vi "START ADD USER.vi"(10 "REFERENCES":T2, 11 "USER INFO IN":T1) -> (2 "User Image":T3, 3 "USER INFO OUT":T1)   [LabVIEW 2019]
uses:
  <vilib>/vision/Image Controls.llb/IMAQ Image.ctl
  Controls/References Cluster.ctl
  <vilib>/userDefined/High Color/IMAQdx.ctl
  Controls/Custom Calendar/Custom Calendar.xctl
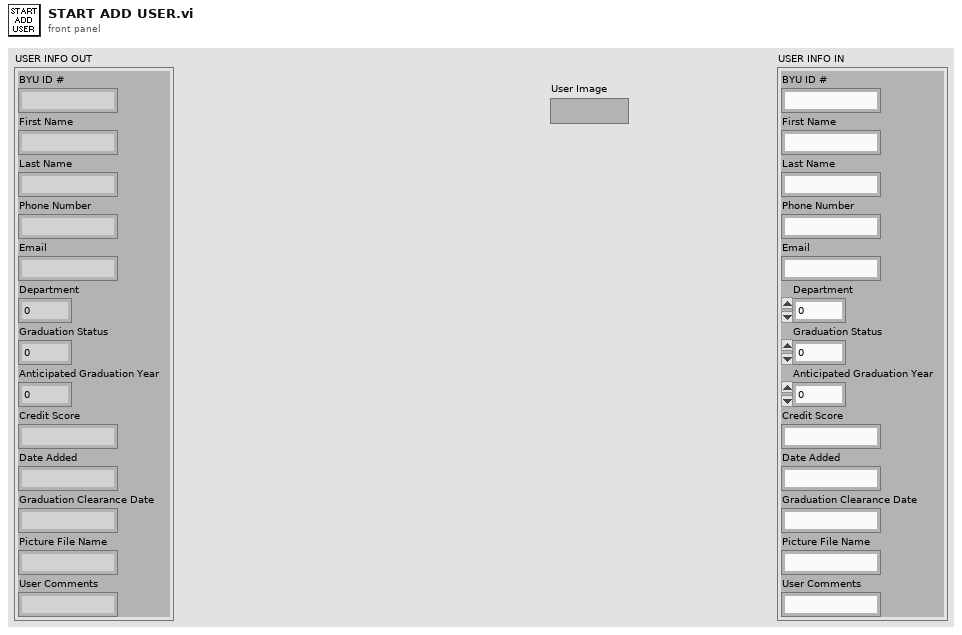
[diagram p1: front panel]
types:
  T1 = cluster{"BYU ID #":string, "First Name":string, "Last Name":string, "Phone Number":string, "Email":string, "Department":u16, "Graduation Status":u16, "Anticipated Graduation Year":u16, "Credit Score":string, "Date Added":string, "Graduation Clearance Date":string, "Picture File Name":string, "User Comments":string}
  T2 = typedef "References Cluster.ctl" = cluster{"MAIN PAGES":refnum<vi>, "ADD/EDIT ITEM REFERENCES":cluster{"Identifier":refnum<vi>, "BYU ICN #":refnum<vi>, "Item Description":refnum<vi>, "Comments":refnum<vi>, "Checked Out Date":refnum<vi>, "Due Date":refnum<vi>, "Check Out Location":refnum<vi>, "Reminder Count":refnum<vi>, "Most Recent Reminder Date":refnum<vi>, "BYU ID #":refnum<vi>, "Building/Room":refnum<vi>, "Location in Room":refnum<vi>, "Manual":refnum<vi>, "Manufacturer":refnum<vi>, "Model #":refnum<vi>, "Serial #":refnum<vi>, "Date Acquired":refnum<vi>, "ADD/EDIT ITEM LABEL":refnum<vi>, "ARCHIVE ITEM":refnum<vi>, "Archive Item Inputs":refnum<vi>, "Reminder Notes":refnum<vi>}, "ADD/EDIT USER REFERENCES":cluster{"BYU ID # (##-###-####)":refnum<vi>, "First Name":refnum<vi>, "Last Name":refnum<vi>, "Phone Number (###-###-####)":refnum<vi>, "Email":refnum<vi>, "Department":refnum<vi>, "Graduation Status":refnum<vi>, "Anticipated Graduation Year":refnum<vi>, "Credit Score":refnum<vi>, "Date Added":refnum<vi>, "Graduation Clearance Date":refnum<vi>, "Picture File Name":refnum<vi>, "ADD/EDIT USER LABEL":refnum<vi>, "Department Map":refnum<vi>, "Status Map":refnum<vi>, "Anticipated Graduation Year Map":refnum<vi>, "User Agreement":refnum<vi>, "User Comments":refnum<vi>, "Camera":refnum<vi>}, "RETURN ITEM REFERENCES":cluster{"Item or Person:":refnum<vi>, "Search Return Results":refnum<vi>, "What are you searching for?":refnum<vi>}, "SEARCH DATABASE REFERENCES":cluster{"What to Search For:":refnum<vi>, "Where to Search":refnum<vi>, "Column to Search In":refnum<vi>, "Column to Sort By":refnum<vi>, "Search Database Results":refnum<vi>, "Inventory Column Selector":refnum<vi>, "User Column Selector":refnum<vi>, "Inventory Archive Column Selector":refnum<vi>, "User Archive Column Selector":refnum<vi>, "Sales Tracking Column Selector":refnum<vi>, "Checked In Archive Column Selector":refnum<vi>, "Restore User":refnum<vi>, "Date Range":refnum<vi>, "Dates Less Than":refnum<vi>, "Dates Greater Than":refnum<vi>, "Search Print Receipt":refnum<vi>}, "USER ITEMS REFERENCES":cluster{"USER'S INFORMATION":refnum<vi>, "User's Checked Out Items":refnum<vi>, "User Info Comments":refnum<vi>, "SEE USER INFO COMMENTS":refnum<vi>}, "EDIT ITEMS REFERENCES":cluster{"New Check Out Location":refnum<vi>, "Items to Edit":refnum<vi>, "Edit Items Due Date":refnum<vi>, "New Reminder Notes":refnum<vi>, "New Item Description":refnum<vi>}, "CHECK OUT ITEMS REFERENCES":cluster{"Enter Item:":refnum<vi>, "Check Out Items Due Date":refnum<vi>, "Check Out Location":refnum<vi>, "Items to be Checked Out":refnum<vi>, "Possible Items":refnum<vi>}, "TRANSFER ITEMS REFERENCES":cluster{"Search Parameter":refnum<vi>, "What to Match":refnum<vi>, "Matching Individuals":refnum<vi>, "Items to be Transferred":refnum<vi>}, "SETTINGS REFERENCES":cluster{"PSC Database Settings":refnum<vi>, "PSC Sales Item Spreadsheet":refnum<vi>}, "PSC SALES REFERENCES":cluster{"BYU ID CARD #":refnum<vi>, "Sale Description":refnum<vi>, "Scan or Enter Item Name":refnum<vi>, "Items to be Sold":refnum<vi>, "Grand Total":refnum<vi>, "Item List":refnum<vi>}}
  T3 = typedef "IMAQ Image.ctl" = refnum<image>
  T4 = typedef "Image Type" = u32
  T5 = enum8{"Enabled", "Disabled", "Disabled and Grayed Out"}
  T6 = enum32{"IDLE", "ADD/EDIT USER", "ADD/EDIT ITEM", "RETURN ITEMS", "SEARCH DATABASE", "USER ITEMS", "CHECK OUT ITEMS", "EDIT ITEMS", "TRANSFER ITEMS", "PSC SALES", "ATRIUM", "INVENTORY TRACKING", "SETTINGS"}
  T7 = cluster{"BYU ID # (##-###-####)":refnum<vi>, "First Name":refnum<vi>, "Last Name":refnum<vi>, "Phone Number (###-###-####)":refnum<vi>, "Email":refnum<vi>, "Department":refnum<vi>, "Graduation Status":refnum<vi>, "Anticipated Graduation Year":refnum<vi>, "Credit Score":refnum<vi>, "Date Added":refnum<vi>, "Graduation Clearance Date":refnum<vi>, "Picture File Name":refnum<vi>, "ADD/EDIT USER LABEL":refnum<vi>, "Department Map":refnum<vi>, "Status Map":refnum<vi>, "Anticipated Graduation Year Map":refnum<vi>, "User Agreement":refnum<vi>, "User Comments":refnum<vi>, "Camera":refnum<vi>}
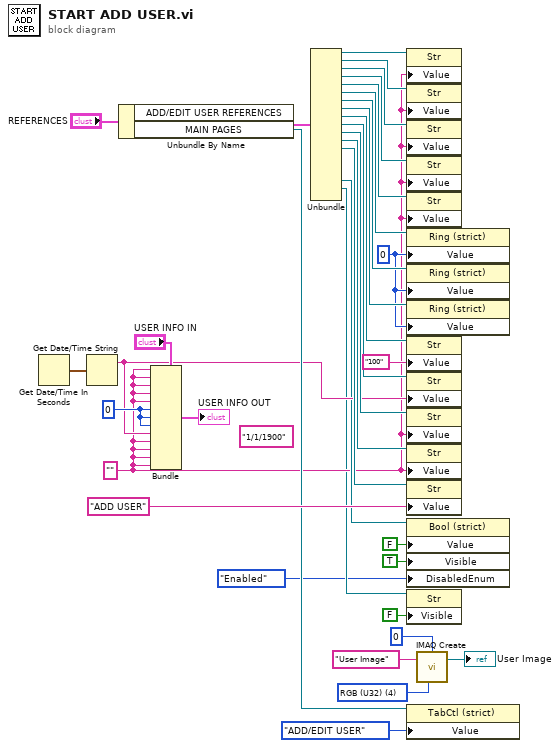
[diagram p0: block diagram]
diagram:
  w2 = T4 4 items=["Grayscale (U8)", "Grayscale (I16)", "Grayscale (SGL)", "Complex (CSG)", "RGB (U32)", "HSL (U32)", "RGB (U64)", "Grayscale (U16)"] ("Image Type")
  (unwired) "1/1/1900" ("Value")
  w20 = u16 0 ("Department")
  w21 = u16 0 ("Value")
  w6 = "" ("Value")
  n1 = Get Date/Time In Seconds() -> (seconds since 1Jan1904=w23:timestamp)
  n2 = Get Date/Time String(seconds (now)=w23) -> (date string=w10:string)  [unwired: 2 in, 1 out]
  n3 = Unbundle By Name("REFERENCES") -> ("ADD/EDIT USER REFERENCES"=w16:T7, "MAIN PAGES"=w13:refnum<vi>)
  n4 = Bundle(cluster="USER INFO IN", "BYU ID #"=w6, "First Name"=w6, "Last Name"=w6, "Phone Number"=w6, "Email"=w6, "Department"=w20, "Graduation Status"=w20, "Anticipated Graduation Year"=w20, "Credit Score"=w10, "Date Added"=w6, "Graduation Clearance Date"=w6, "Picture File Name"=w6, "User Comments"=w6) -> (→"USER INFO OUT":T1)
  n5 = Unbundle(w16) -> ("BYU ID # (##-###-####)"=w36:refnum<vi>, "First Name"=w35:refnum<vi>, "Last Name"=w34:refnum<vi>, "Phone Number (###-###-####)"=w33:refnum<vi>, "Email"=w32:refnum<vi>, "Department"=w31:refnum<vi>, "Graduation Status"=w30:refnum<vi>, "Anticipated Graduation Year"=w29:refnum<vi>, "Credit Score"=w28:refnum<vi>, "Date Added"=w27:refnum<vi>, "Graduation Clearance Date"=w26:refnum<vi>, "Picture File Name"=w25:refnum<vi>, "ADD/EDIT USER LABEL"=w24:refnum<vi>, "User Agreement"=w9:refnum<vi>, "User Comments"=w5:refnum<vi>)  [unwired: 4 out]
  n6 = property class="Str"(reference=w36, "Value"=w6) -> ()  [unwired: 1 in, 2 out]
  n7 = property class="Str"(reference=w35, "Value"=w6) -> ()  [unwired: 1 in, 2 out]
  n8 = property class="Str"(reference=w34, "Value"=w6) -> ()  [unwired: 1 in, 2 out]
  n9 = property class="Str"(reference=w33, "Value"=w6) -> ()  [unwired: 1 in, 2 out]
  n10 = property class="Str"(reference=w32, "Value"=w6) -> ()  [unwired: 1 in, 2 out]
  n11 = property class="Ring (strict)"(reference=w31, "Value"=w21) -> ()  [unwired: 1 in, 2 out]
  n12 = property class="Ring (strict)"(reference=w30, "Value"=w21) -> ()  [unwired: 1 in, 2 out]
  n13 = property class="Ring (strict)"(reference=w29, "Value"=w21) -> ()  [unwired: 1 in, 2 out]
  n14 = property class="Str"(reference=w28, "Value"="100") -> ()  [unwired: 1 in, 2 out]
  n15 = property class="Str"(reference=w27, "Value"=w10) -> ()  [unwired: 1 in, 2 out]
  n16 = property class="Str"(reference=w26, "Value"=w6) -> ()  [unwired: 1 in, 2 out]
  n17 = property class="Str"(reference=w25, "Value"=w6) -> ()  [unwired: 1 in, 2 out]
  n18 = property class="Str"(reference=w24, "Value"="ADD USER") -> ()  [unwired: 1 in, 2 out]
  n19 = property class="Bool (strict)"(reference=w9, "Value"=FALSE, "Visible"=TRUE, "DisabledEnum"=T5."Enabled" ("Disabled")) -> ()  [unwired: 1 in, 2 out]
  n20 = property class="Str"(reference=w5, "Visible"=FALSE) -> ()  [unwired: 1 in, 2 out]
  n21 = property class="TabCtl (strict)"(reference=w13, "Value"=T6."ADD/EDIT USER") -> ()  [unwired: 1 in, 2 out]
  n22 = call "IMAQ Create"("Border Size"=0, "Image Name"="User Image", "Image Type"=w2) -> ("New Image"=→"User Image":T3)  [unwired: 2 in, 1 out]
